vi "Insert Plugin.vi"(8 "error in":errorcluster, 9 "vi path":path=path "Plugins/Plugin - Splash.vi", 10 "Message Queues":T1, 11 "SubPanel in":refnum<vi>) -> (0 "error out":errorcluster, 3 "SubPanel out":refnum<vi>)   [LabVIEW 2019]
uses:
  support/Copy of Message Queue/All Message Queues.ctl
  support/Copy of Message Queue/Message Cluster.ctl
  support/Copy of Message Queue/Copy of Message Queue.lvlib
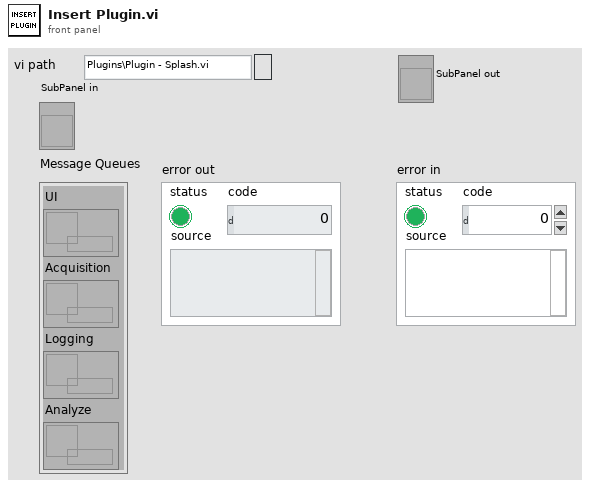
[diagram p1: front panel]
types:
  T1 = typedef "Copy of Message Queue.lvlib/All Message Queues.ctl" = cluster{"UI":refnum<queue>, "Acquisition":refnum<queue>, "Logging":refnum<queue>, "Analyze":refnum<queue>}
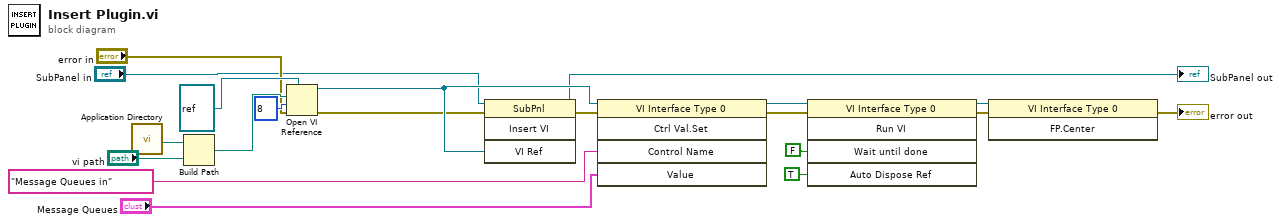
[diagram p0: block diagram]
diagram:
  n1 = call <vilib>:"Application Directory.vi"() -> ("Application Directory"=w6:path)
  n2 = Build Path(base path=w6, name or relative path="vi path") -> (appended path=w8:path)
  n3 = Open VI Reference(type specifier VI Refnum (for type only)=refnum<vi> refnum ("reference out"), vi path=w8, options=8, error in (no error)="error in") -> (vi reference=w15:refnum<vi>, error out=w1:errorcluster)  [unwired: 2 in]
  n4 = invoke on="Invoke Node" class="SubPnl" method="Insert VI"(reference="SubPanel in", error in=w1, "VI Ref"=w15) -> (reference out=→"SubPanel out":refnum<vi>, error out=w16:errorcluster)  [unwired: 1 in, 2 out]
  n5 = invoke class="VI Interface Type 0" method="Ctrl Val.Set"(reference=w15, error in=w16, "Control Name"="Message Queues in", "Value"="Message Queues") -> (reference out=w17:refnum<vi>, error out=w20:errorcluster)  [unwired: 1 in, 3 out]
  n6 = invoke class="VI Interface Type 0" method="Run VI"(reference=w17, error in=w20, "Wait until done"=FALSE ("Wait Until Done"), "Auto Dispose Ref"=TRUE ("Wait Until Done")) -> (reference out=w18:refnum<vi>, error out=w19:errorcluster)  [unwired: 1 in, 3 out]
  n7 = invoke class="VI Interface Type 0" method="FP.Center"(reference=w18, error in=w19) -> (error out=→"error out":errorcluster)  [unwired: 1 in, 2 out]
